vi "onProcessStart.vi"(8 "error in (no error)":errorcluster, 11 "EmbeddedMainUI":refnum<class "EmbeddedMainUI.lvclass">) -> (0 "error out":errorcluster, 3 "EmbeddedMainUI out":refnum<class "EmbeddedMainUI.lvclass">)   [LabVIEW 2016, in "EmbeddedMainUI.lvclass"]
doc: "JKI State Machine Objects (SMO) 1.3.0.56\nJKI - JKI\nCopyright (c) 2017, JKI"
uses:
  EmbeddedMainUI.lvclass
  <vilib>/Levylab/Embedded SMO UI/EmbeddedSMO.lvclass
  C:/Program Files (x86)/National Instruments/LabVIEW 2016/vi.lib/JKI/JKI SMO/SMO/SMO.lvclass
  <vilib>/JKI/JKI SMO/SMO.UI/SMO.UI.lvclass
  <vilib>/JKI/JKI SMO/SMO/SMO.lvclass
panel:
  # "For instructions on how to use the JKI State Machine Objects, examples and video tutorials, visit:\nhttp://jki.net/state-machine-objects/\n\nJKI State Machine Objects™\nhttp://jki.net/state-machine-objects/\nCopyright (C) 2005-2015, JKI <info@jki.net>\nALL RIGHTS RESERVED"
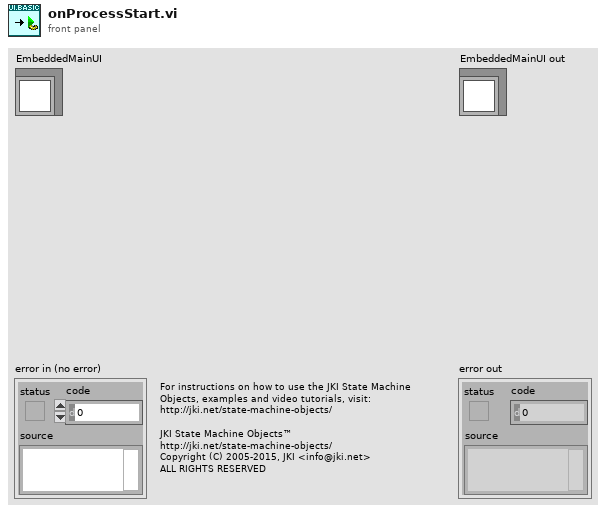
[diagram p1: front panel]
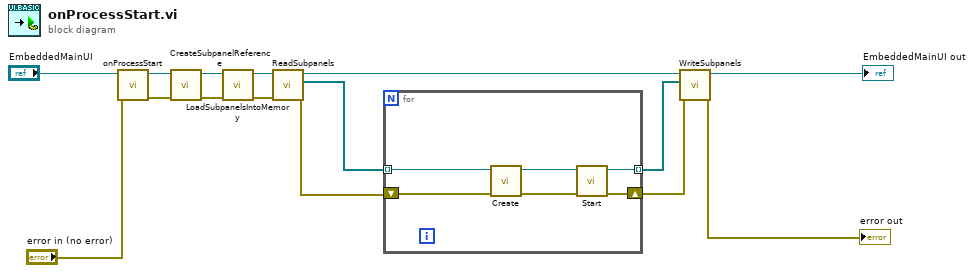
[diagram p0: block diagram]
diagram:
  n1 = call-parent "onProcessStart.vi"("error in (no error)"="error in (no error)", "SMO"="EmbeddedMainUI") -> ("error out"=w10:errorcluster, "SMO out"=w13:refnum<class "EmbeddedMainUI.lvclass">)  [unwired: 8 in]
  n2 = call "CreateSubpanelReference.vi"("error in (no error)"=w10, "EmbeddedMainUI in"=w13) -> ("error out"=w11:errorcluster, "EmbeddedMainUI out"=w12:refnum<class "EmbeddedMainUI.lvclass">)  [unwired: 8 in]
  n3 = call "LoadSubpanelsIntoMemory.vi"("error in (no error)"=w11, "EmbeddedMainUI in"=w12) -> ("error out"=w6:errorcluster, "EmbeddedMainUI out"=w9:refnum<class "EmbeddedMainUI.lvclass">)  [unwired: 8 in]
  n4 = call "ReadSubpanels.vi"("error in (no error)"=w6, "EmbeddedMainUI in"=w9) -> ("error out"=w7:errorcluster, "Subpanels"=w8:refnum<class "EmbeddedSMO.lvclass">[], "EmbeddedMainUI out"=w5:refnum<class "EmbeddedMainUI.lvclass">)  [unwired: 7 in]
  n5 = for {
    tunnel: w8 -> [w17] mode=indexing
    shift-right: [w19] -> w2
    shift-left: w7 -> [w16]
    tunnel: [w18] -> w3 mode=indexing
    n6 = call <vilib>:"Create.vi"("error in (no error)"=w16, "SMO"=w17) -> ("error out"=w20:errorcluster, "SMO out"=w21:refnum<class "EmbeddedSMO.lvclass">)  [unwired: 7 in, 1 out]
    n7 = call <vilib>:"Start.vi"("error in (no error)"=w20, "SMO"=w21) -> ("error out"=w19:errorcluster, "SMO out"=w18:refnum<class "EmbeddedSMO.lvclass">)  [unwired: 8 in]
  }
  n8 = call "WriteSubpanels.vi"("error in (no error)"=w2, "Subpanels"=w3, "EmbeddedMainUI in"=w5) -> ("error out"=→"error out":errorcluster, "EmbeddedMainUI out"=→"EmbeddedMainUI out":refnum<class "EmbeddedMainUI.lvclass">)  [unwired: 7 in]
